vi "SearchForErrors.vi"(0 "DTC (ASCII)":string[][](table), 5 "error in (no error)":errorcluster) -> (13 "DTC codes (error)":string[](array[string]), 14 "DTC info out":T1(array[cluster]), 15 "Scrap?":bool, 16 "ERROR?":bool, 17 "Only DTC errors":string, 18 "Logging output":string, 19 "error out":errorcluster)   [LabVIEW 2012]
panel:
  out "Conversion for report AUDI (copy + paste to Excel)":string
  out "size(s)":i32[](array[numeric])
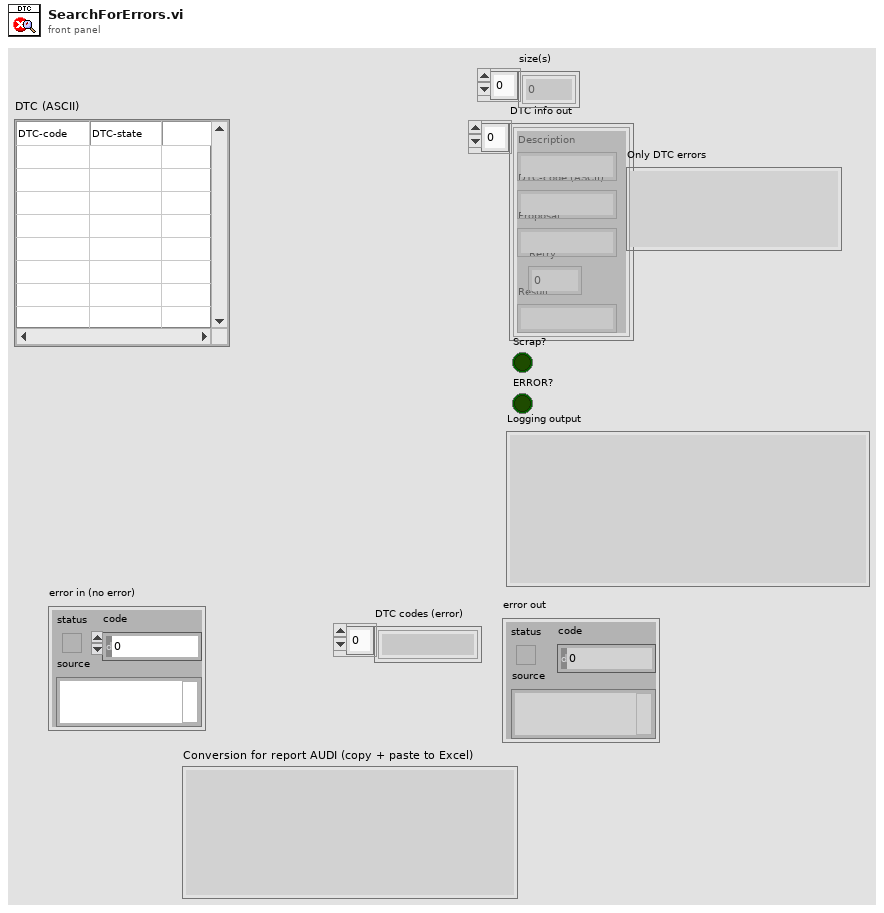
[diagram p1: front panel]
types:
  T1 = cluster{"Description":string, "DTC-code (ASCII)":string, "Proposal":string, "Retry":i32, "Result":string}[]
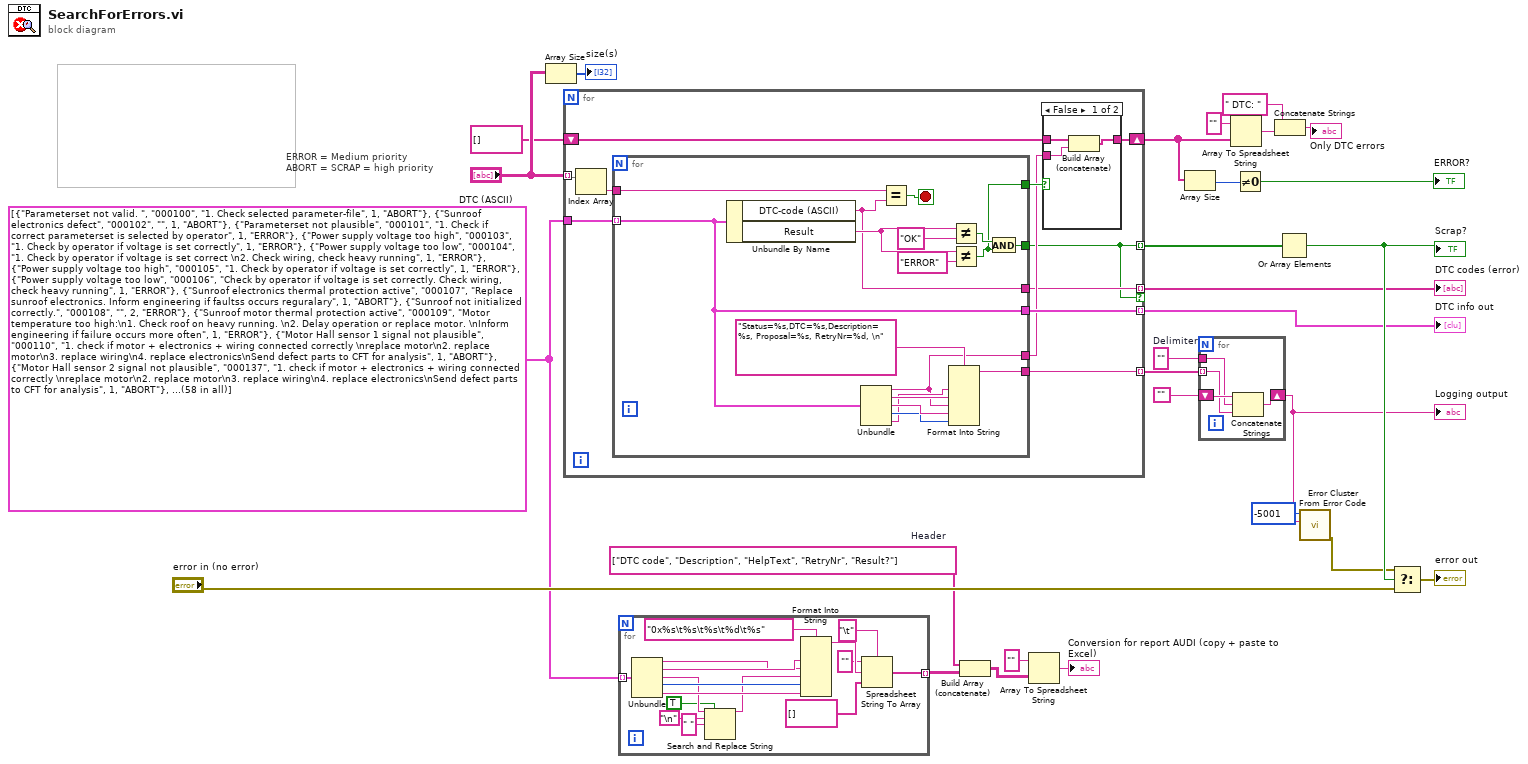
[diagram p0: block diagram]
diagram:
  w12 = string[] ["DTC code", "Description", "HelpText", "RetryNr", "Result?"]  # Header
  w21 = ""  # Delimiter
  w16 = T1 [{"Description"="Parameterset not valid. ", "DTC-code (ASCII)"="000100", "Proposal"="1. Check selected parameter-file", "Retry"=1, "Result"="ABORT"}, {"Description"="Sunroof electronics defect", "DTC-code (ASCII)"="000102", "Proposal"="", "Retry"=1, "Result"="ABORT"}, {"Description"="Parameterset not plausible", "DTC-code (ASCII)"="000101", "Proposal"="1. Check if correct parameterset is selected by operator", "Retry"=1, "Result"="ERROR"}, {"Description"="Power supply voltage too high", "DTC-code (ASCII)"="000103", "Proposal"="1. Check by operator if voltage is set correctly", "Retry"=1, "Result"="ERROR"}, {"Description"="Power supply voltage too low", "DTC-code (ASCII)"="000104", "Proposal"="1. Check by operator if voltage is set correct \n2. Check wiring, check heavy running", "Retry"=1, "Result"="ERROR"}, {"Description"="Power supply voltage too high", "DTC-code (ASCII)"="000105", "Proposal"="1. Check by operator if voltage is set correctly", "Retry"=1, "Result"="ERROR"}, {"Description"="Power supply voltage too low", "DTC-code (ASCII)"="000106", "Proposal"="Check by operator if voltage is set correctly. Check wiring, check heavy running", "Retry"=1, "Result"="ERROR"}, {"Description"="Sunroof electronics thermal protection active", "DTC-code (ASCII)"="000107", "Proposal"="Replace sunroof electronics. Inform engineering if faultss occurs reguralary", "Retry"=1, "Result"="ABORT"}, {"Description"="Sunroof not initialized correctly.", "DTC-code (ASCII)"="000108", "Proposal"="", "Retry"=2, "Result"="ERROR"}, {"Description"="Sunroof motor thermal protection active", "DTC-code (ASCII)"="000109", "Proposal"="Motor temperature too high:\n1. Check roof on heavy running. \n2. Delay operation or replace motor. \nInform engineering if failure occurs more often", "Retry"=1, "Result"="ERROR"}, {"Description"="Motor Hall sensor 1 signal not plausible", "DTC-code (ASCII)"="000110", "Proposal"="1. check if motor + electronics + wiring connected correctly \nreplace motor\n2. replace motor\n3. replace wiring\n4. replace electronics\nSend defect parts to CFT for analysis", "Retry"=1, "Result"="ABORT"}, {"Description"="Motor Hall sensor 2 signal not plausible", "DTC-code (ASCII)"="000137", "Proposal"="1. check if motor + electronics + wiring connected correctly \nreplace motor\n2. replace motor\n3. replace wiring\n4. replace electronics\nSend defect parts to CFT for analysis", "Retry"=1, "Result"="ABORT"}, {"Description"="Hall sensor signal short circuit to ground", "DTC-code (ASCII)"="000138", "Proposal"="Check and replace modules:\n1. Motor\n2. Wiring\n3. Electronics", "Retry"=1, "Result"="ABORT"}, {"Description"="Hall sensor signal short circuit to plus", "DTC-code (ASCII)"="000139", "Proposal"="Check and replace modules:\n1. Motor\n2. Wiring\n3. Electronics", "Retry"=1, "Result"="ABORT"}, {"Description"="Short circuit to ground", "DTC-code (ASCII)"="000111", "Proposal"="Check and replace modules:\n1. Motor\n2. Wiring\n3. Electronics", "Retry"=1, "Result"="ABORT"}, {"Description"="Short circuit to battery plus", "DTC-code (ASCII)"="000140", "Proposal"="Check and replace modules:\n1. Motor\n2. Wiring\n3. Electronics", "Retry"=1, "Result"="ABORT"}, {"Description"="Rollo not initialized correctly.", "DTC-code (ASCII)"="000112", "Proposal"="", "Retry"=2, "Result"="ERROR"}, {"Description"="Rollo motor thermal protection active", "DTC-code (ASCII)"="000113", "Proposal"="Motor temperature too high:\n1. Check roof on heavy running. \n2. Delay operation or replace motor. \nInform engineering if failures occurs more often", "Retry"=1, "Result"="ABORT"}, {"Description"="Motor Rollo Hall sensor 1 signal not plausible", "DTC-code (ASCII)"="000114", "Proposal"="1. check if motor + electronics + wiring connected correctly \nreplace motor\n2. replace motor\n3. replace wiring\n4. replace electronics\nSend defect parts to CFT for analysis", "Retry"=1, "Result"="ABORT"}, {"Description"="Motor Rollo Hall sensor 2 signal not plausible", "DTC-code (ASCII)"="000141", "Proposal"="1. check if motor + electronics + wiring connected correctly \nreplace motor\n2. replace motor\n3. replace wiring\n4. replace electronics\nSend defect parts to CFT for analysis", "Retry"=1, "Result"="ABORT"}, {"Description"="Hall sensor Rollo signal short circuit to ground", "DTC-code (ASCII)"="000142", "Proposal"="Check and replace modules:\n1. Motor\n2. Wiring\n3. Electronics", "Retry"=1, "Result"="ABORT"}, {"Description"="Hall sensor Rollo signal short circuit to plus", "DTC-code (ASCII)"="000143", "Proposal"="Check and replace modules:\n1. Motor\n2. Wiring\n3. Electronics", "Retry"=1, "Result"="ABORT"}, {"Description"="Rollo Short circuit to ground", "DTC-code (ASCII)"="000115", "Proposal"="Check and replace modules:\n1. Motor\n2. Wiring\n3. Electronics", "Retry"=1, "Result"="ABORT"}, {"Description"="Rollo Short circuit to battery plus", "DTC-code (ASCII)"="000144", "Proposal"="Check and replace modules:\n1. Motor\n2. Wiring\n3. Electronics", "Retry"=1, "Result"="ABORT"}, {"Description"="Inplausible signal received for tilt open/close", "DTC-code (ASCII)"="000116", "Proposal"="1. Check if connected correclty. \n2. Check switch module. \n3. Check and replace module", "Retry"=1, "Result"="ABORT"}, {"Description"="Inplausible signal received for slide open/close", "DTC-code (ASCII)"="000117", "Proposal"="1. Check if connected correclty. \n2. Check switch module. \n3. Check and replace module", "Retry"=1, "Result"="ABORT"}, {"Description"="Sunroof Switch tilt open close button mechanical problem", "DTC-code (ASCII)"="000118", "Proposal"="Check switch module", "Retry"=1, "Result"="ABORT"}, {"Description"="Sunroof Switch slide open close button mechanical problem", "DTC-code (ASCII)"="000119", "Proposal"="Check switch module", "Retry"=1, "Result"="ABORT"}, {"Description"="Rollo Switch tilt open close button mechanical problem", "DTC-code (ASCII)"="000120", "Proposal"="Check switch module", "Retry"=1, "Result"="ABORT"}, {"Description"="Rollo Switch slide open close button mechanical problem", "DTC-code (ASCII)"="000121", "Proposal"="Check switch module", "Retry"=1, "Result"="ABORT"}, {"Description"="Switch lightning signal short circuit to ground", "DTC-code (ASCII)"="000122", "Proposal"="Check and replace wiring", "Retry"=1, "Result"="ABORT"}, {"Description"="Switch lightning signal short circuit to battery plus", "DTC-code (ASCII)"="000123", "Proposal"="Check and replace wiring", "Retry"=1, "Result"="ABORT"}, {"Description"="Switch lightning signal short circuit to ground", "DTC-code (ASCII)"="000124", "Proposal"="Check and replace wiring", "Retry"=1, "Result"="ABORT"}, {"Description"="Switch lightning signal short circuit to battery plus", "DTC-code (ASCII)"="000125", "Proposal"="Check and replace wiring", "Retry"=1, "Result"="ABORT"}, {"Description"="Production mode is activated", "DTC-code (ASCII)"="000126", "Proposal"="", "Retry"=1, "Result"="OK"}, {"Description"="No signal received from PXI", "DTC-code (ASCII)"="000127", "Proposal"="Check connection to test station", "Retry"=1, "Result"="ABORT"}, {"Description"="No signal received from PXI", "DTC-code (ASCII)"="000128", "Proposal"="Check connection to test station", "Retry"=1, "Result"="ABORT"}, {"Description"="No signal received from PXI", "DTC-code (ASCII)"="000129", "Proposal"="Check connection to test station", "Retry"=1, "Result"="ABORT"}, {"Description"="No signal received from PXI", "DTC-code (ASCII)"="000130", "Proposal"="Check connection to test station", "Retry"=1, "Result"="ABORT"}, {"Description"="No signal received from PXI", "DTC-code (ASCII)"="000131", "Proposal"="Check connection to test station", "Retry"=1, "Result"="ABORT"}, {"Description"="No signal received from PXI", "DTC-code (ASCII)"="000149", "Proposal"="Check connection to test station", "Retry"=1, "Result"="ABORT"}, {"Description"="No signal received from PXI", "DTC-code (ASCII)"="000150", "Proposal"="Check connection to test station", "Retry"=1, "Result"="ABORT"}, {"Description"="No signal received from PXI", "DTC-code (ASCII)"="000132", "Proposal"="Check connection to test station", "Retry"=1, "Result"="ABORT"}, {"Description"="No signal received from PXI", "DTC-code (ASCII)"="000133", "Proposal"="Check connection to test station", "Retry"=1, "Result"="ABORT"}, {"Description"="No signal received from PXI", "DTC-code (ASCII)"="000134", "Proposal"="Check connection to test station", "Retry"=1, "Result"="ABORT"}, {"Description"="No signal received from PXI", "DTC-code (ASCII)"="000135", "Proposal"="Check connection to test station", "Retry"=1, "Result"="ABORT"}, {"Description"="Engineering modus active in Electronics SW", "DTC-code (ASCII)"="000136", "Proposal"="", "Retry"=1, "Result"="OK"}, {"Description"="No vehicle type coded", "DTC-code (ASCII)"="000145", "Proposal"="", "Retry"=2, "Result"="ABORT"}, {"Description"="Incorrect parameterset", "DTC-code (ASCII)"="000147", "Proposal"="Retry flashing (2x)\nor replace electronics", "Retry"=1, "Result"="ABORT"}, {"Description"="CAN transceiver failure on electronics", "DTC-code (ASCII)"="000148", "Proposal"="Replace electronics", "Retry"=1, "Result"="ABORT"}, {"Description"="Electronics not initialized correctly.", "DTC-code (ASCII)"="000151", "Proposal"="Repeat initialization (2x)", "Retry"=2, "Result"="ERROR"}, {"Description"="Electronics not initialized correctly.", "DTC-code (ASCII)"="000152", "Proposal"="Repeat initialization (2x)", "Retry"=1, "Result"="ERROR"}, {"Description"="Flash modus active", "DTC-code (ASCII)"="000153", "Proposal"="", "Retry"=1, "Result"="OK"}, {"Description"="Incorrect signal received from PXI", "DTC-code (ASCII)"="000154", "Proposal"="Check connection to test station", "Retry"=1, "Result"="ABORT"}, {"Description"="Incorrect signal received from PXI", "DTC-code (ASCII)"="000155", "Proposal"="Check connection to test station", "Retry"=1, "Result"="ABORT"}, {"Description"="Incorrect signal received from PXI", "DTC-code (ASCII)"="000156", "Proposal"="Check connection to test station", "Retry"=1, "Result"="ABORT"}, {"Description"="Incorrect signal received from PXI", "DTC-code (ASCII)"="000157", "Proposal"="Check connection to test station", "Retry"=1, "Result"="ABORT"}, {"Description"="Undefined", "DTC-code (ASCII)"="Undefined", "Proposal"="Undefined", "Retry"=1, "Result"="Undefined"}]
  # "ERROR = Medium priority\nABORT = SCRAP = high priority"
  n1 = Array Size(array="DTC (ASCII)") -> (size(s)=→"size(s)":i32[])
  n2 = for {
    tunnel: "DTC (ASCII)" -> [w38] mode=indexing
    tunnel: w16 -> [w39]
    tunnel: [w36] -> w10 mode=indexing
    tunnel: [w29] -> w28 mode=indexing
    tunnel: [w33] -> w20 mode=indexing
    shift-right: [w32] -> w6
    shift-left: string[] [] ("DTC (ASCII)") -> [w34]
    tunnel: [w30] -> w1 mode=indexing if=w29
    n3 = Index Array(array=w38) -> (element=w37:string)  [unwired: 1 in]
    n4 = for {
      tunnel: w39 -> [w57] mode=indexing
      tunnel: w37 -> [w60]
      tunnel: [w57] -> w36
      tunnel: [w48] -> w29
      tunnel: [w55] -> w33
      tunnel: [w46] -> w35
      tunnel: [w45] -> w31
      tunnel: [w44] -> w30
      stop <- w59 stop-if-true
      n5 = Unbundle By Name(w57) -> ("DTC-code (ASCII)"=w44:string, "Result"=w47:string)
      n6 = Unbundle(w57) -> ("Description"=w45:string, "DTC-code (ASCII)"=w52:string, "Proposal"=w54:string, "Retry"=w53:i32, "Result"=w51:string)
      n7 = Equal?(x=w60, y=w44) -> (x = y?=w59:bool)
      n8 = Format Into String(format string="Status=%s,DTC=%s,Description= %s, Proposal=%s, RetryNr=%d, \n", w51, w52, w45, w54, w53) -> (resulting string=w55:string)  [unwired: 2 in, 1 out]
      n9 = Not Equal?(x=w47, y="OK") -> (x != y?=w50:bool)
      n10 = Not Equal?(x=w47, y="ERROR") -> (x != y?=w46:bool)
      n11 = And(x=w50, y=w46) -> (x .and. y?=w48:bool)
    }
    n12 = case shown="False" w35 {
      tunnel: w34 -> [w42 w43]
      tunnel: w31 -> [w41 _]
      tunnel: [w40 w43] -> w32
      frame False {
        n13 = Build Array (concatenate)(w42, w41) -> (w40:string[])
      }
      frame True {
      }
    }
  }
  "DTC info out" <- w10
  "DTC codes (error)" <- w1
  n14 = for {
    tunnel: w16 -> [w76] mode=indexing
    tunnel: [w67] -> w13 mode=indexing
    n15 = Unbundle(w76) -> ("Description"=w71:string, "DTC-code (ASCII)"=w72:string, "Proposal"=w65:string, "Retry"=w75:i32, "Result"=w74:string)
    n16 = Search and Replace String(replace all?=TRUE ("replace all? (F)"), input string=w65, search string="\n", replace string=" " ("replace string (\"\")")) -> (result string=w61:string)  [unwired: 4 in, 3 out]
    n17 = Format Into String(format string="0x%s\t%s\t%s\t%d\t%s", w72, w71, w61, w75, w74) -> (resulting string=w70:string)  [unwired: 2 in, 1 out]
    n18 = Spreadsheet String To Array(delimiter (Tab)="\t", format string="", spreadsheet string=w70, array type (2D Dbl)=string[] []) -> (array=w67:string[])
  }
  n19 = Build Array (concatenate)(w12, w13) -> (w11:string[][])
  n20 = Array To Spreadsheet String(array=w11, 3:"" ("format string")) -> (spreadsheet string=→"Conversion for report AUDI (copy + paste to Excel)":string)  [unwired: 1 in]
  n21 = Array Size(array=w6) -> (size(s)=w8:i32)
  n22 = for {
    tunnel: w20 -> [w79] mode=indexing
    shift-right: [w78] -> w19
    shift-left: "" -> [w80]
    tunnel: w21 -> [w77]
    n23 = Concatenate Strings(w80, w77, w79) -> (w78:string)
  }
  "Logging output" <- w19
  n24 = Array To Spreadsheet String(array=w6, 3:"" ("format string")) -> (spreadsheet string=w4:string)  [unwired: 1 in]
  n25 = Not Equal To 0?(x=w8) -> (x != 0?=→"ERROR?":bool)
  n26 = Concatenate Strings(" DTC: " ("string"), w4) -> (→"Only DTC errors":string)
  n27 = Or Array Elements(Boolean array=w28) -> (logical OR=w26:bool)
  "Scrap?" <- w26
  n28 = call <vilib>:"Error Cluster From Error Code.vi"("error message (\"\")"=w19, "error code (0)"=-5001) -> ("error out"=w25:errorcluster)  [unwired: 7 in]
  n29 = Select(t=w25, s=w26, f="error in (no error)") -> (s? t:f=→"error out":errorcluster)
